vi "Process.vi"(8 "error in":errorcluster, 11 "StreamReader":refnum<class "StreamReader.lvclass">) -> (0 "error out":errorcluster, 3 "StreamReader out":refnum<class "StreamReader.lvclass">)   [LabVIEW 2016, in "StreamReader.lvclass"]
doc: "---------------------------------------------------------------\nJKI State Machine Objects™\nhttp://jki.net/state-machine-objects/\nCopyright (C) 2005-2015, JKI <info@jki.net>\nALL RIGHTS RESERVED"
uses:
  StreamReader.lvclass
  C:/Program Files/National Instruments/LabVIEW 2016/vi.lib/JKI/JKI SMO/SMO/SMO.lvclass
  <vilib>/JKI/JKI SMO/SMO/Typedefs/Parent Call--Enum.ctl
  <vilib>/JKI/JKI SMO/SMO/SMO.lvclass
  <resource>/objmgr/ni.dex.rc
panel:
  in  "start":bool
  in  "stop":bool
  out "full URL":string
  in  "Target IP Address":string="localhost"
  out "Signals Graph":waveform(dbl)[](graph)=[{"t0"=timestamp(3565974471.4961195 s since 1904-01-01), "dt"=1.0, "Y"=array[6023 elements], "attributes"=variant("NI_ChannelName"=variant(string "Dev2/ai0"), "NI_UnitDescription"=variant(string "Volts"))}, {"t0"=timestamp(3565974471.4961195 s since 1904-01-01), "dt"=1.0, "Y"=array[6023 elements], "attributes"=variant("NI_ChannelName"=variant(string "Dev2/ai1"), "NI_UnitDescription"=variant(string "Volts"))}, {"t0"=timestamp(3565974471.4961195 s since 1904-01-01), "dt"=1.0, "Y"=array[6023 elements], "attributes"=variant("NI_ChannelName"=variant(string "Dev2/ai2"), "NI_UnitDescription"=variant(string "Volts"))}, {"t0"=timestamp(3565974471.4961195 s since 1904-01-01), "dt"=1.0, "Y"=array[6023 elements], "attributes"=variant("NI_ChannelName"=variant(string "Dev2/ai3"), "NI_UnitDescription"=variant(string "Volts"))}, {"t0"=timestamp(3565974471.554943 s since 1904-01-01), "dt"=1.0, "Y"=array[6023 elements], "attributes"=variant("NI_ChannelName"=variant(string "Dev2/ai0"), "NI_UnitDescription"=variant(string "Volts"))}, {"t0"=timestamp(3565974471.554943 s since 1904-01-01), "dt"=1.0, "Y"=array[6023 elements], "attributes"=variant("NI_ChannelName"=variant(string "Dev2/ai1"), "NI_UnitDescription"=variant(string "Volts"))}]
  out "Available Elements to Read":i32
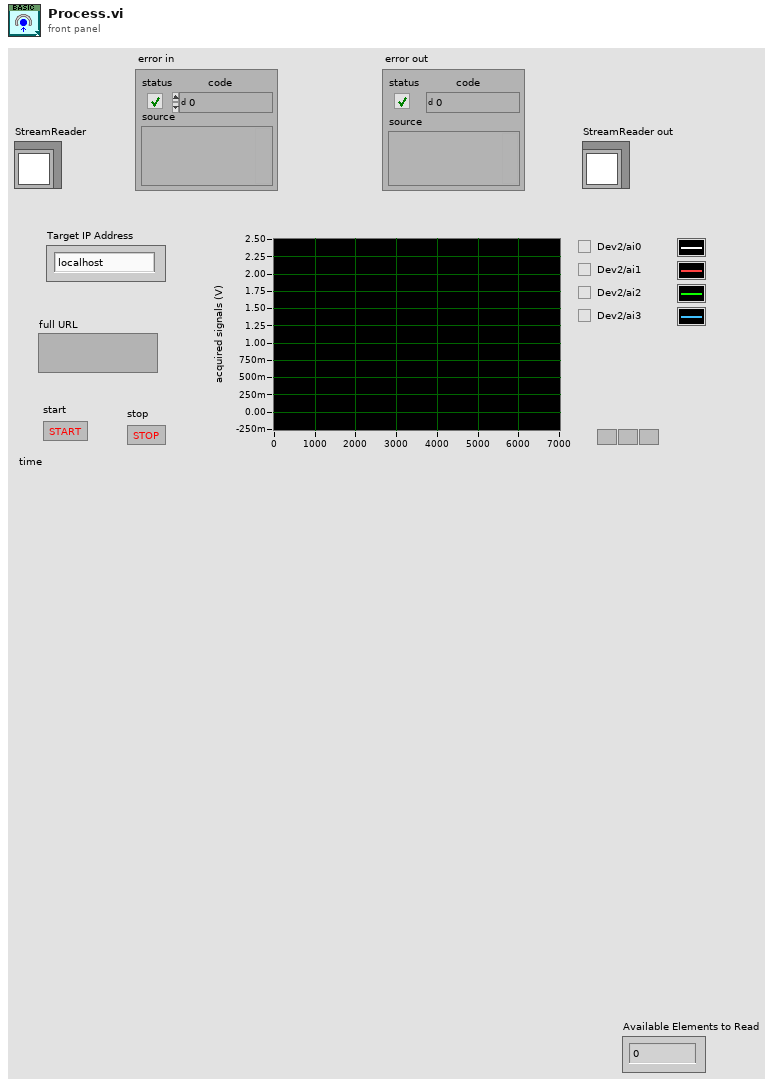
[diagram p1: front panel]
types:
  T1 = typedef "SMO.lvclass/Parent Call--Enum.ctl" = enum16{"Allows parent to run", "Does not request parent to run"}
  T2 = enum32{"invalid app kind", "Development System", "Run Time System", "Student Edition", "Embedded LabVIEW", "Evaluation", "Custom"}
  T3 = enum32{"Invalid", "Standard", "Closed", "Hidden", "Minimized", "Maximized"}
  T4 = enum32{"Bad", "Idle", "Run top level", "Running"}
  T5 = cluster{"Core":cluster{"Current VI Reference":refnum<vi>, "Close Panel on Exit?":bool, "error":errorcluster}, "Self Reference":refnum<class "StreamReader.lvclass">, "Your string data":string, "reader endpoint":refnum<k21>}
  T6 = cluster{"Current VI Reference":refnum<vi>, "Close Panel on Exit?":bool, "error":errorcluster}
  T7 = typedef "SMO.lvclass/Protected Events.ctl" = cluster{"StopProcesses":refnum<user-event>, "AbortProcesses":refnum<user-event>, "Config Changed":refnum<user-event>, "Dependency":refnum<user-event>}
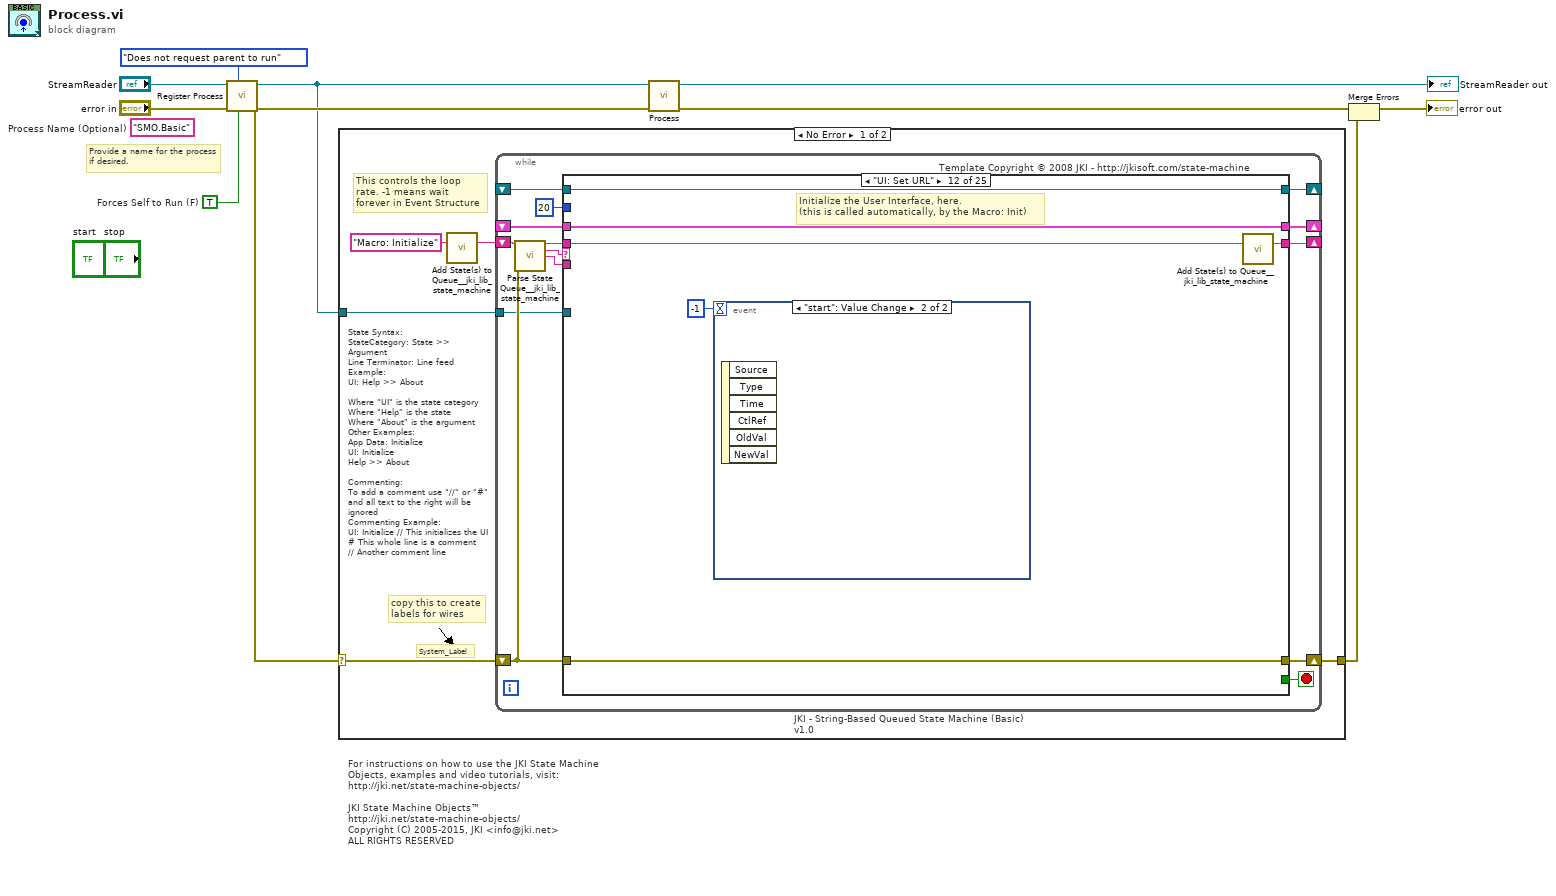
[diagram p0: block diagram]
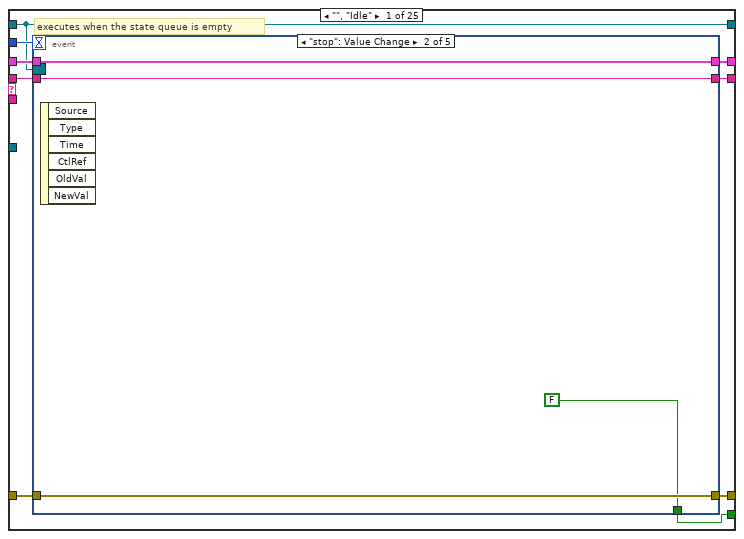
[diagram p2: hidden frame]
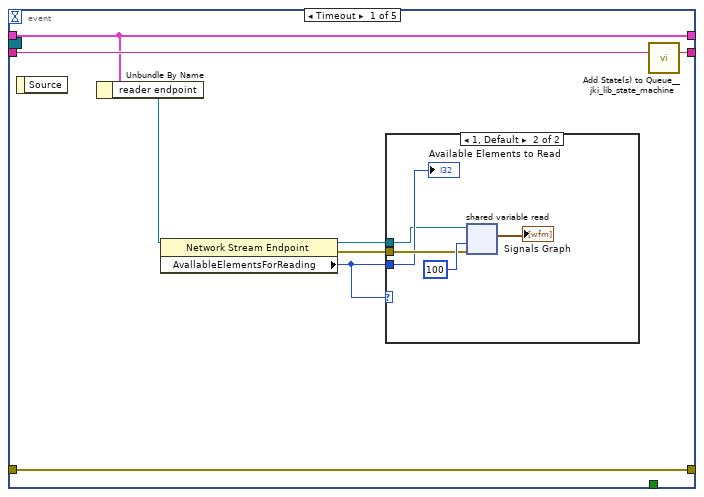
[diagram p3: hidden frame]
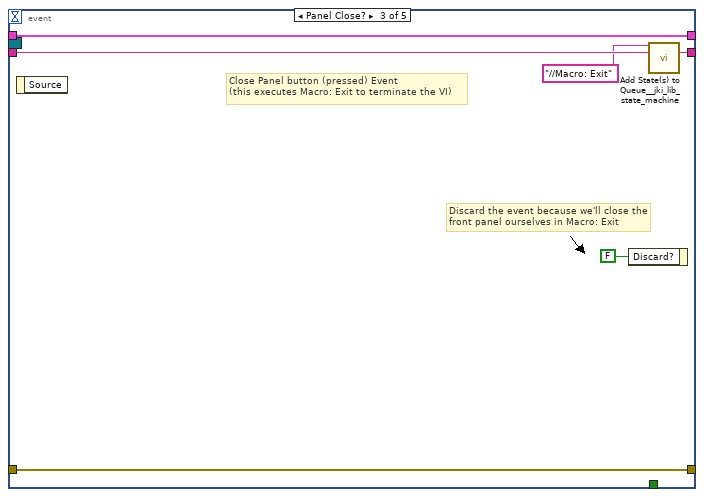
[diagram p5: hidden frame]
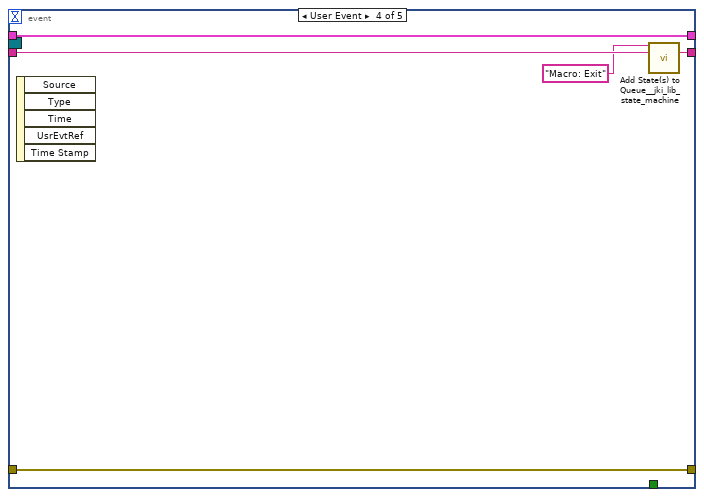
[diagram p6: hidden frame]
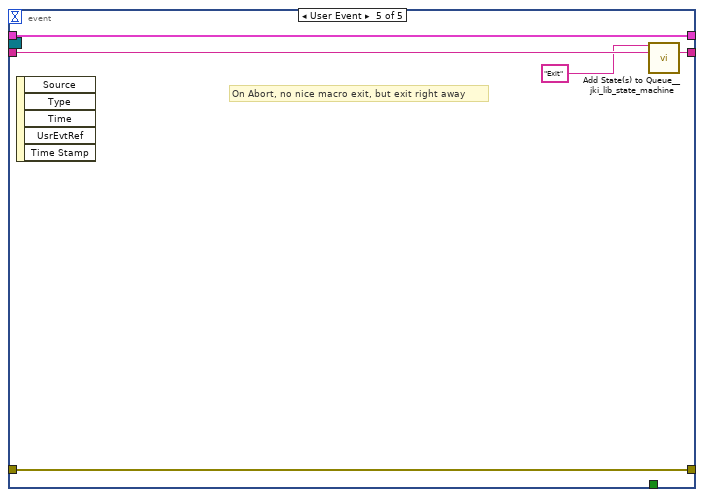
[diagram p7: hidden frame]
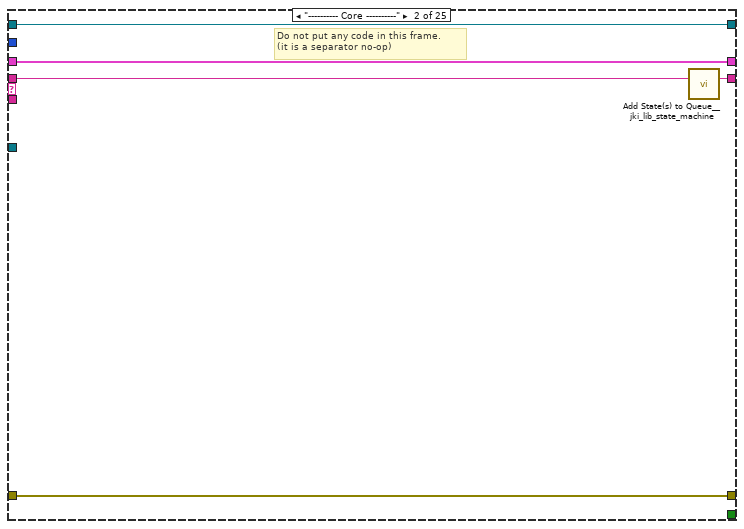
[diagram p8: hidden frame]
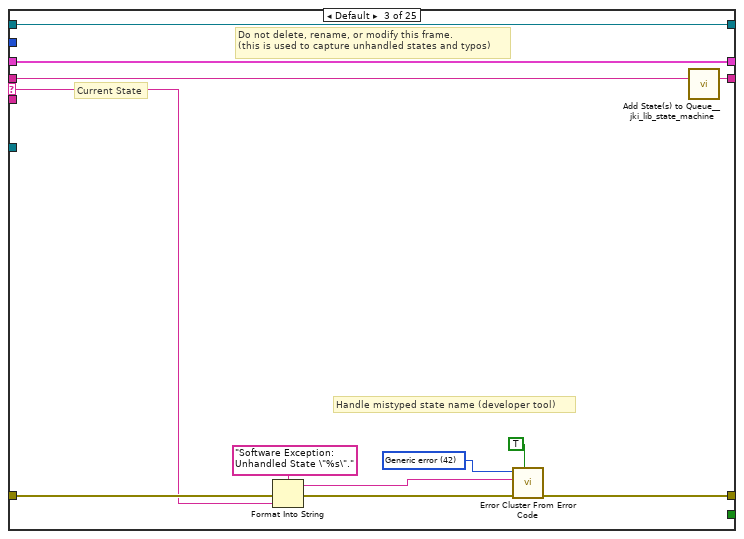
[diagram p9: hidden frame]
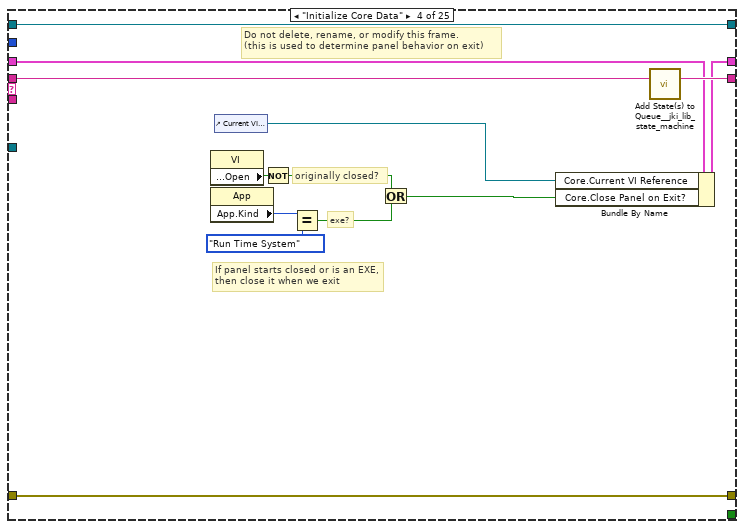
[diagram p10: hidden frame]
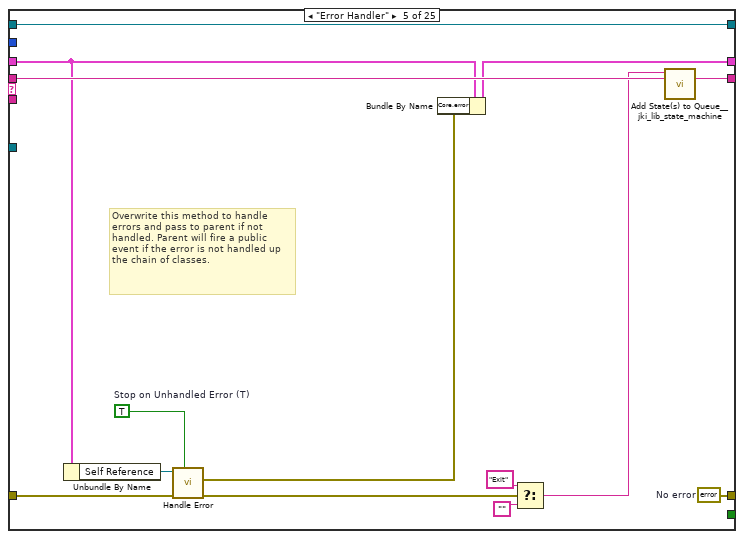
[diagram p11: hidden frame]
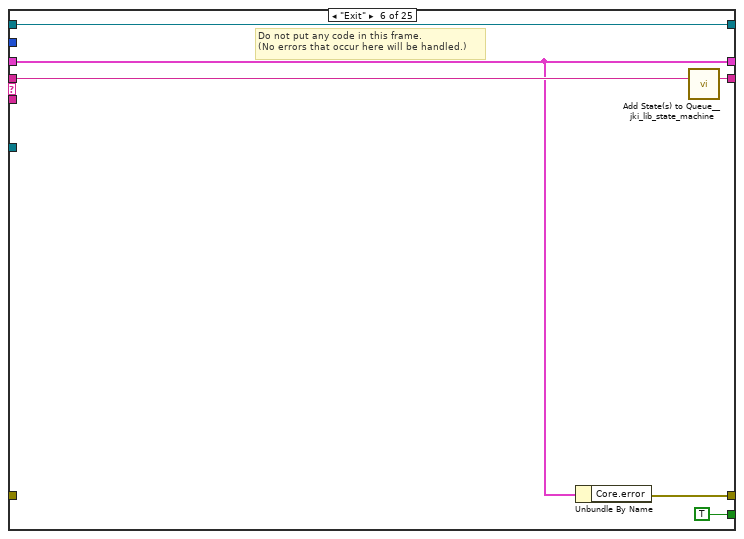
[diagram p12: hidden frame]
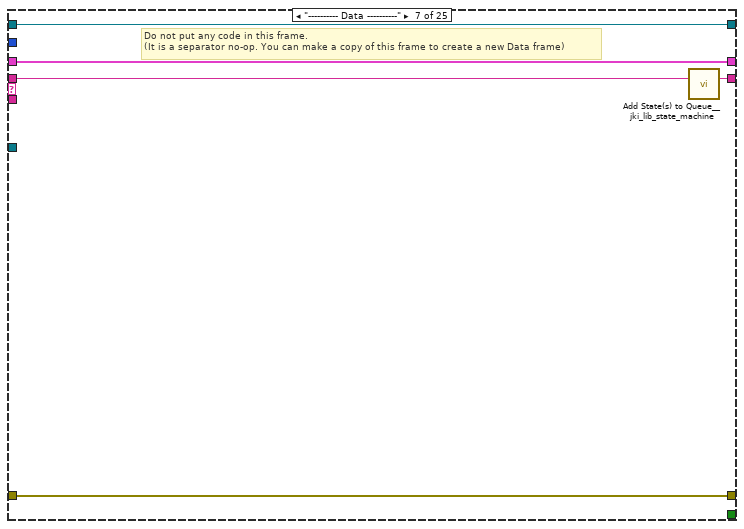
[diagram p13: hidden frame]
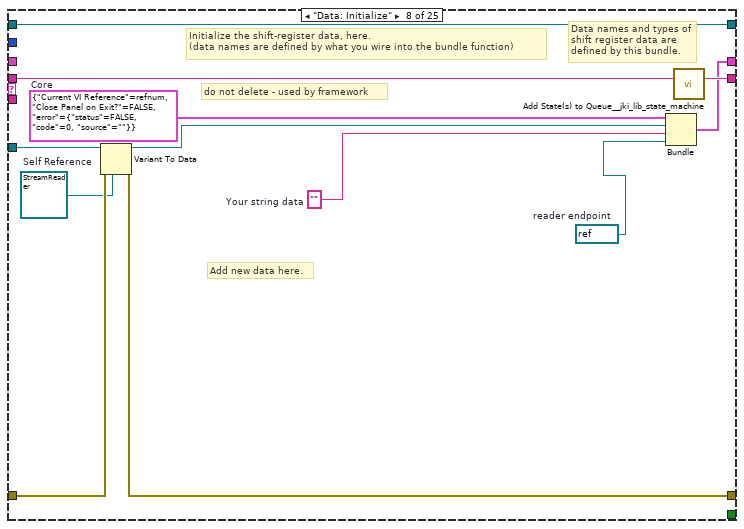
[diagram p14: hidden frame]
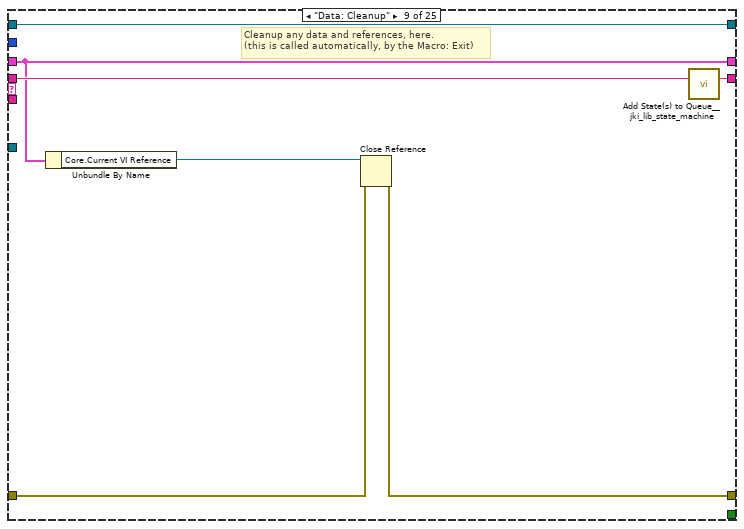
[diagram p15: hidden frame]
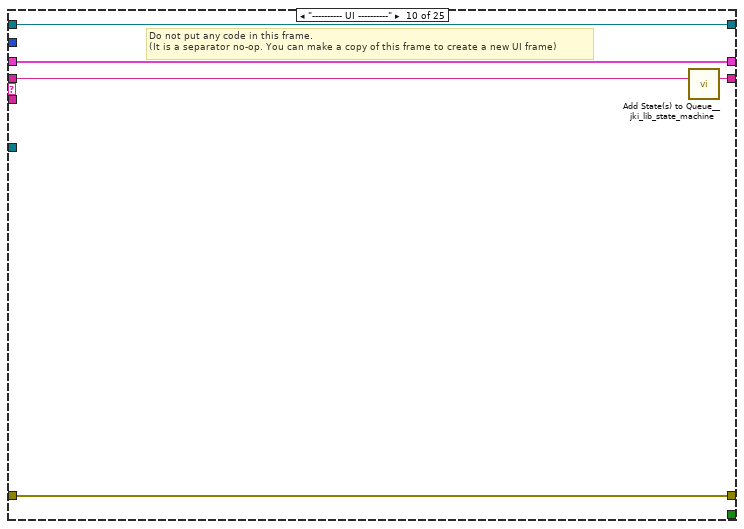
[diagram p16: hidden frame]
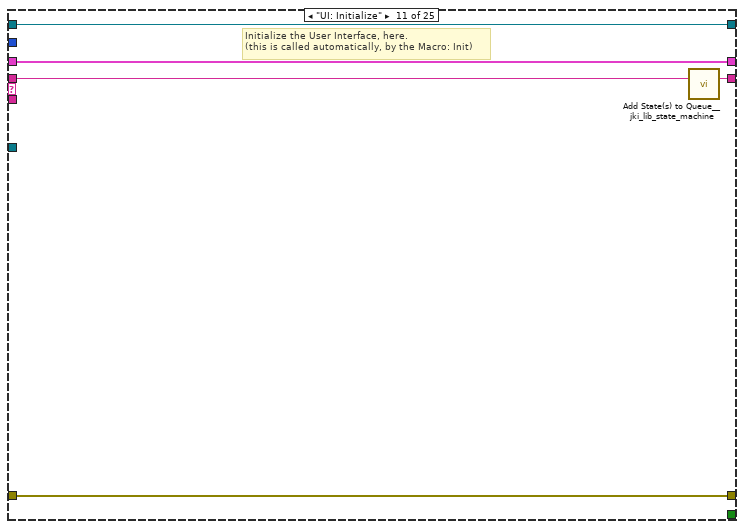
[diagram p17: hidden frame]
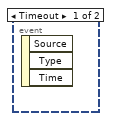
[diagram p18: hidden frame]
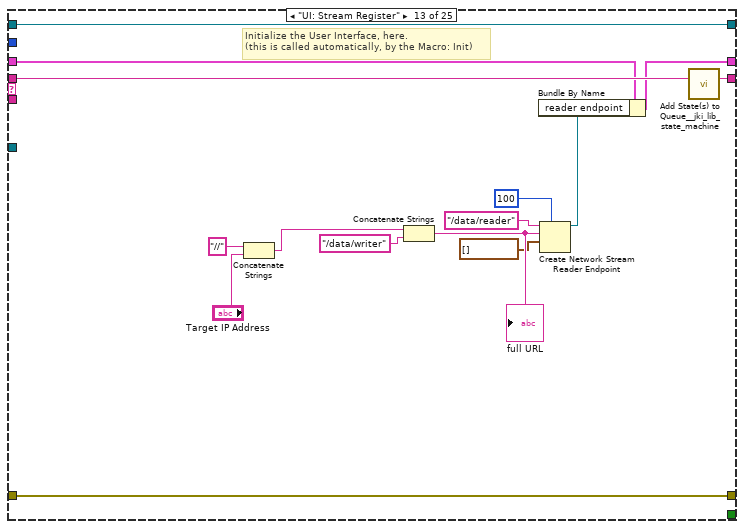
[diagram p19: hidden frame]
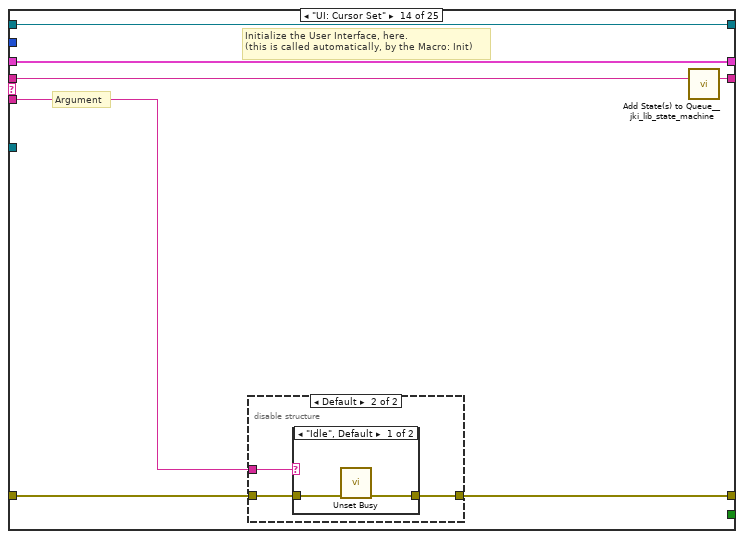
[diagram p20: hidden frame]
diagram:
  w1 = TRUE  # Forces Self to Run (F)
  (unwired) "SMO.Basic"  # Process Name (Optional)
  # "Provide a name for the process\nif desired."
  # "For instructions on how to use the JKI State Machine Objects, examples and video tutorials, visit:\nhttp://jki.net/state-machine-objects/\n\nJKI State Machine Objects™\nhttp://jki.net/state-machine-objects/\nCopyright (C) 2005-2015, JKI <info@jki.net>\nALL RIGHTS RESERVED"
  n1 = call <vilib>:"Register Process.vi"("Forces Self to Run (F)"=w1, "Parent Call"=Parent_Call--Enum."Does not request parent to run", "error in (no error)"="error in", "SMO"="StreamReader") -> ("error out"=w7:errorcluster, "SMO out"=w6:refnum<class "StreamReader.lvclass">)  [unwired: 6 in]
  n2 = case shown="No Error" w7 {
    selector: w7 -> [w12 w310]
    tunnel: w6 -> [w13 _]
    tunnel: [w11 w310] -> w3
    frame No Error {
      # "State Syntax:\nStateCategory: State >> Argument\nLine Terminator: Line feed\nExample:\nUI: Help >> About\n\nWhere \"UI\" is the state category\nWhere \"Help\" is the state\nWhere \"About\" is the argument\nOther Examples:\nApp Data: Initialize\nUI: Initialize\nHelp >> About\n\nCommenting:\nTo add a comment use \"//\" or \"#\" and all text to the right will be ignored\nCommenting Example:\nUI: Initialize // This initializes the UI\n# This whole line is a comment\n// Another comment line"
      # "copy this to create labels for wires"
      # "This controls the loop rate. -1 means wait forever in Event Structure"
      # "System_Label"
      n3 = call <vilib>:"Add State(s) to Queue__jki_lib_state_machine.vi"("State(s) in (\"\")"="Macro: Initialize") -> ("States Out"=w15:string)  [unwired: 14 in]
      n4 = while "JKI - String-Based Queued State Machine (Basic) v1.0" {
        shift-right: [w22] -> _
        shift-left: _ -> [w21]
        shift-right: [w25] -> w11
        shift-left: w12 -> [w19]
        shift-right: [w24] -> _
        shift-left: w15 -> [w26]
        tunnel: w13 -> [w18]
        shift-right: [w17] -> _
        shift-left: _ -> [w16]
        stop <- w23 stop-if-true
        # "Template Copyright © 2008 JKI - http://jkisoft.com/state-machine"
        n5 = call <vilib>:"Parse State Queue__jki_lib_state_machine.vi"("State Queue"=w26, "Error In (no error)"=w19) -> ("Remaining States"=w28:string, "Current State"=w29:string, "Arguments"=w27:string)  [unwired: 11 in]
        n6 = case shown="\"UI: Set URL\"" w29 {
          selector: w29 -> [_ _ w78 _ _ _ _ _ _ _ _ _ _ _ _ _ _ _ _ _ _ _ _ _ _]
          tunnel: w28 -> [w38 w76 w82 w101 w115 w121 w126 w138 w145 w150 w155 w161 w176 w183 w199 w231 w245 w260 w265 w276 w281 w291 w297 w302 w309]
          tunnel: w27 -> [_ _ _ _ _ _ _ _ _ _ _ _ _ w177 w193 _ _ _ _ _ _ _ _ _ _]
          tunnel: w21 -> [w36 w73 w80 w92 w109 w117 w123 _ w140 w147 w151 w157 w166 w181 w195 w228 w241 w251 w262 w273 w278 w289 w295 w300 w305]
          tunnel: [w35 w74 w84 w98 w110 w116 w124 w133 w141 w148 w153 w159 w174 w178 w196 w229 w243 w258 w263 w267 w279 w284 w293 w298 w306] -> w25
          tunnel: w19 -> [w34 w74 w83 w98 w111 _ w124 w134 w142 w148 w153 w159 w174 w179 w197 w229 w243 w258 w263 w268 w279 w285 w293 w298 w306]
          tunnel: [w37 w75 w81 w100 w114 w120 w125 w137 w144 w149 w154 w160 w175 w182 w198 w230 w244 w259 w264 w275 w280 w290 w296 w301 w308] -> w24
          tunnel: [w30 _ _ _ _ TRUE _ _ _ _ _ _ _ _ _ _ _ _ _ _ _ _ _ _ _] -> w23
          tunnel: [w33 w73 w80 w99 w108 w117 w123 w136 w140 w147 w151 w157 w165 w181 w195 w228 w241 w251 w262 w273 w278 w289 w295 w300 w304] -> w22
          tunnel: 20 ("Timeout") -> [w32 _ _ _ _ _ _ _ _ _ _ _ _ _ _ _ _ _ _ _ _ _ _ _ _]
          tunnel: w18 -> [_ _ _ _ _ _ _ w131 _ _ _ _ _ _ _ _ _ _ _ _ _ _ _ _ _]
          tunnel: [w31 w72 w77 w89 w113 w118 w122 w129 w139 w146 w152 w158 w173 w180 w192 w227 w242 w252 w261 w274 w277 w288 w294 w299 w307] -> w17
          tunnel: w16 -> [w31 w72 w77 w89 w113 w118 w122 w129 w139 w146 w152 w158 w173 w180 w192 w227 w242 w252 w261 w274 w277 _ w294 w299 w307]
          frame "", "Idle" {
            # "executes when the state queue is empty"
            n7 = event shown="[1] \"stop\": Value Change" {
              selector: w31 -> [_ _ _ _ _]
              dyn-events: _ -> [_ _ _ _ _]
              timeout: w32 -> [_ _ _ _ _]
              tunnel: w38 -> [w46 w53 w61 w66 w71]
              tunnel: [w45 w53 w60 w65 w70] -> w37
              tunnel: w36 -> [w41 w54 w58 w63 w68]
              tunnel: [w44 w55 w59 w64 w69] -> w35
              tunnel: w34 -> [w44 w55 w59 w64 w69]
              tunnel: [w41 w54 w58 w63 w68] -> w33
              tunnel: [_ FALSE _ _ _] -> w30
              event Timeout {
                n8 = event-data() -> ()  [unwired: 1 in, 1 out]
                n9 = Unbundle By Name(w41) -> ("reader endpoint"=w40:refnum<k21>)
                n10 = property class="Network Stream Endpoint"(reference=w40) -> (reference out=w42:refnum<k21>, error out=w43:errorcluster, "AvallableElementsForReading"=w39:i32)  [unwired: 1 in]
                n11 = case shown="1, Default" w39 {
                  tunnel: w43 -> [_ w50]
                  tunnel: w39 -> [_ w49]
                  tunnel: w42 -> [_ w47]
                  frame 0 {
                  }
                  frame 1, Default {
                    n12 = shared-variable-read(w47, w50, 100 ("timeout ms")) -> (→"Signals Graph":waveform(dbl)[])  [unwired: 3 out]
                    "Available Elements to Read" <- w49
                  }
                }
                n13 = call <vilib>:"Add State(s) to Queue__jki_lib_state_machine.vi"("State(s) in (\"\")"=w46) -> ("States Out"=w45:string)  [unwired: 14 in]
              }
              event "stop": Value Change {
                n14 = event-data() -> ()  [unwired: 1 in, 6 out]
              }
              event Panel Close? {
                # "Discard the event because we'll close the front panel ourselves in Macro: Exit"
                # "Close Panel button (pressed) Event\n(this executes Macro: Exit to terminate the VI)"
                n15 = event-data() -> ()  [unwired: 1 in, 1 out]
                n16 = event-data("Discard?"=FALSE) -> ()  [unwired: 1 in, 1 out]
                n17 = call <vilib>:"Add State(s) to Queue__jki_lib_state_machine.vi"("State(s) in Front (\"\")"="//Macro: Exit", "State(s) in (\"\")"=w61) -> ("States Out"=w60:string)  [unwired: 13 in]
              }
              event User Event {
                n18 = event-data() -> ()  [unwired: 1 in, 5 out]
                n19 = call <vilib>:"Add State(s) to Queue__jki_lib_state_machine.vi"("State(s) in Front (\"\")"="Macro: Exit", "State(s) in (\"\")"=w66) -> ("States Out"=w65:string)  [unwired: 13 in]
              }
              event User Event {
                # "On Abort, no nice macro exit, but exit right away"
                n20 = event-data() -> ()  [unwired: 1 in, 5 out]
                n21 = call <vilib>:"Add State(s) to Queue__jki_lib_state_machine.vi"("State(s) in Front (\"\")"="Exit", "State(s) in (\"\")"=w71) -> ("States Out"=w70:string)  [unwired: 13 in]
              }
            }
          }
          frame "---------- Core ----------" {
            # "Do not put any code in this frame.\n(it is a separator no-op)"
            n22 = call <vilib>:"Add State(s) to Queue__jki_lib_state_machine.vi"("State(s) in (\"\")"=w76) -> ("States Out"=w75:string)  [unwired: 14 in]
          }
          frame Default {
            w87 = 42 items=["No error", "Argument error", "Memory is full", "Out of zone", "End of file", "File already open", "Generic file I/O error", "File not found", "File permission error", "Disk is full", "Duplicate path", "Too many files open", "System feature not enabled", "Resource file not found", "Cannot add resource", "Resource not found", "Image not found", "Image memory error", "Pen does not exist", "Config type invalid", "Config token not found", "Config parse error", "Config memory error", "Bad external code format", "Bad external code offset", "External code not present", "Null window", "Destroy window error", "Null menu", "Print aborted", "Bad print record", "Print driver error", "Windows error during printing", "Memory error during printing", "Print dialog error", "Generic print error", "Invalid device refnum", "Device not found", "Device parameter error", "Device unit error", "Cannot open device", "Device call aborted", "Generic error", "Cancelled by user", "Object ID too low", "Object ID too high", "Object not in heap", "Unknown heap", "Unknown object (invalid DefProc)", "Unknown object (DefProc not in table)", "Message out of range", "Invalid (null) method", "Unknown message", "Manager call not supported", "Bad address", "Network operation in progress", "Network operation timed out", "Connection is busy", "Network attribute not supported", "Network error", "Address in use", "System out of memory", "Connection aborted", "Connection refused", "Not connected", "Already connected", "Connection closed", "Initialization error (interapplication manager)", "Bad occurrence", "Wait on unbound occurrence handler", "Occurrence queue overflow", "Datalog type conflict", "Unused", "Unrecognized type (interapplication manager)", "Memory corrupt", "Failed to make temporary DLL", "Old CIN version", "Drag socket not found", "Failed to load drop-object", "Failed to register OLE object", "Failed to release OLE object", "Format specifier type mismatch", "Unknown format specifier", "Too few format specifiers", "Too many format specifiers", "Scan failed", "Newer CIN version", "Error converting to variant", "Runtime menu error", "Password tampered", "Variant attribute not found", "Incompatible variant data type", "Event data is not available", "Event Store is not present", "Occurrence is not found", "Event Queue is not created", "Event info is not available", "Refnum passed is NULL", "Error retrieving Class GUID", "Error retrieving CoClass GUID", "Error retrieving TypeLib GUID.", "Bad built application magic bytes.", "Specific driver is different from the specific driver associated with the Logical Name.", "There is no session opened to the class driver.", "Max Error", "MAX - Error with config objects", "MAX - Error loading configuration", "MAX - Group not supported"]
            # "Current State"
            # "Do not delete, rename, or modify this frame.\n(this is used to capture unhandled states and typos)"
            # "Handle mistyped state name (developer tool)"
            n23 = Format Into String(format string="Software Exception: Unhandled State \"%s\"." ("message"), error in=w83, w78) -> (resulting string=w86:string, error out=w85:errorcluster)  [unwired: 1 in]
            n24 = call <vilib>:"Error Cluster From Error Code.vi"("show call chain? (False)"=TRUE, "error in (no error)"=w85, "error message (\"\")"=w86, "error code (0)"=w87) -> ("error out"=w84:errorcluster)  [unwired: 5 in]
            n25 = call <vilib>:"Add State(s) to Queue__jki_lib_state_machine.vi"("State(s) in (\"\")"=w82) -> ("States Out"=w81:string)  [unwired: 14 in]
          }
          frame "Initialize Core Data" {
            # "Do not delete, rename, or modify this frame.\n(this is used to determine panel behavior on exit)"
            # "originally closed?"
            # "exe?"
            # "If panel starts closed or is an EXE, then close it when we exit"
            n26 = property class="VI"() -> ("Front Panel.Open"=w97:bool)  [unwired: 2 in, 2 out]
            n27 = property class="App"() -> ("App.Kind"=w96:T2)  [unwired: 2 in, 2 out]
            n28 = control-ref of="Current VI Reference"() -> (w90:refnum<vi>)
            n29 = Not(x=w97) -> (.not. x?=w94:bool)
            n30 = Equal?(x=w96, y=T2."Run Time System" ("Application:Kind")) -> (x = y?=w93:bool)
            n31 = Or(x=w94, y=w93) -> (x .or. y?=w91:bool)
            n32 = Bundle By Name(cluster=w92, "Core.Current VI Reference"=w90, "Core.Close Panel on Exit?"=w91) -> (w99:T5)
            n33 = call <vilib>:"Add State(s) to Queue__jki_lib_state_machine.vi"("State(s) in (\"\")"=w101) -> ("States Out"=w100:string)  [unwired: 14 in]
          }
          frame "Error Handler" {
            w102 = TRUE  # Stop on Unhandled Error (T)
            w110 = errorcluster {"status"=FALSE, "code"=0, "source"=""}  # No error
            # "Overwrite this method to handle errors and pass to parent if not handled. Parent will fire a public event if the error is not handled up the chain of classes."
            n34 = Unbundle By Name(w109) -> ("Self Reference"=w112:refnum<class "StreamReader.lvclass">)
            n35 = call-dynamic "Handle Error.vi"("Stop on Unhandled Error (T)"=w102, "error in"=w111, "SMO"=w112) -> ("handling error"=w103:errorcluster, "Unhandled error"=w106:errorcluster)  [unwired: 6 in, 1 out]
            n36 = Bundle By Name(cluster=w109, "Core.error"=w106) -> (w108:T5)
            n37 = Select(t="Exit", s=w103, f="") -> (s? t:f=w107:string)
            n38 = call <vilib>:"Add State(s) to Queue__jki_lib_state_machine.vi"("State(s) in Front (\"\")"=w107, "State(s) in (\"\")"=w115) -> ("States Out"=w114:string)  [unwired: 13 in]
          }
          frame "Exit" {
            # "Do not put any code in this frame.\n(No errors that occur here will be handled.)"
            n39 = Unbundle By Name(w117) -> ("Core.error"=w116:errorcluster)
            n40 = call <vilib>:"Add State(s) to Queue__jki_lib_state_machine.vi"("State(s) in (\"\")"=w121) -> ("States Out"=w120:string)  [unwired: 14 in]
          }
          frame "---------- Data ----------" {
            # "Do not put any code in this frame.\n(It is a separator no-op. You can make a copy of this frame to create a new Data frame)"
            n41 = call <vilib>:"Add State(s) to Queue__jki_lib_state_machine.vi"("State(s) in (\"\")"=w126) -> ("States Out"=w125:string)  [unwired: 14 in]
          }
          frame "Data: Initialize" {
            w127 = refnum<k21> refnum  # reader endpoint
            w128 = T6 {"Current VI Reference"=refnum, "Close Panel on Exit?"=FALSE, "error"={"status"=FALSE, "code"=0, "source"=""}}  # Core
            w132 = refnum<class "StreamReader.lvclass"> refnum  # Self Reference
            w135 = ""  # Your string data
            # "do not delete - used by framework"
            # "Add new data here."
            # "Data names and types of shift register data are defined by this bundle."
            # "Initialize the shift-register data, here.\n(data names are defined by what you wire into the bundle function)"
            n42 = Variant To Data(error in=w134, type=w132, Variant=w131) -> (data=w130:refnum<class "StreamReader.lvclass">, error out=w133:errorcluster)
            n43 = Bundle("Core"=w128, "Self Reference"=w130, "Your string data"=w135, "reader endpoint"=w127) -> (w136:T5)  [unwired: 1 in]
            n44 = call <vilib>:"Add State(s) to Queue__jki_lib_state_machine.vi"("State(s) in (\"\")"=w138) -> ("States Out"=w137:string)  [unwired: 14 in]
          }
          frame "Data: Cleanup" {
            # "Cleanup any data and references, here.\n(this is called automatically, by the Macro: Exit)"
            n45 = Unbundle By Name(w140) -> ("Core.Current VI Reference"=w143:refnum<vi>)
            n46 = Close Reference(reference=w143, error in (no error)=w142) -> (error out=w141:errorcluster)
            n47 = call <vilib>:"Add State(s) to Queue__jki_lib_state_machine.vi"("State(s) in (\"\")"=w145) -> ("States Out"=w144:string)  [unwired: 14 in]
          }
          frame "---------- UI ----------" {
            # "Do not put any code in this frame.\n(It is a separator no-op. You can make a copy of this frame to create a new UI frame)"
            n48 = call <vilib>:"Add State(s) to Queue__jki_lib_state_machine.vi"("State(s) in (\"\")"=w150) -> ("States Out"=w149:string)  [unwired: 14 in]
          }
          frame "UI: Initialize" {
            # "Initialize the User Interface, here.\n(this is called automatically, by the Macro: Init)"
            n49 = call <vilib>:"Add State(s) to Queue__jki_lib_state_machine.vi"("State(s) in (\"\")"=w155) -> ("States Out"=w154:string)  [unwired: 14 in]
          }
          frame "UI: Set URL" {
            # "Initialize the User Interface, here.\n(this is called automatically, by the Macro: Init)"
            n50 = event shown="[1] \"start\": Value Change" {
              selector: _ -> [_ _]
              dyn-events: _ -> [_ _]
              timeout: -1 -> [_ _]
              event Timeout {
                n51 = event-data() -> ()  [unwired: 1 in, 3 out]
              }
              event "start": Value Change {
                n52 = event-data() -> ()  [unwired: 1 in, 6 out]
              }
            }
            n53 = call <vilib>:"Add State(s) to Queue__jki_lib_state_machine.vi"("State(s) in (\"\")"=w161) -> ("States Out"=w160:string)  [unwired: 14 in]
          }
          frame "UI: Stream Register" {
            # "Initialize the User Interface, here.\n(this is called automatically, by the Macro: Init)"
            n54 = Concatenate Strings("//" ("reader url"), "Target IP Address") -> (w162:string)
            n55 = Concatenate Strings(w162, "/data/writer" ("reader url")) -> (w170:string)
            "full URL" <- w170
            n56 = Create Network Stream Reader Endpoint(7:100 ("reader buffer size"), 9:waveform(dbl)[] [], 10:w170, 11:"/data/reader" ("writer name")) -> (3:w167:refnum<k21>)  [unwired: 3 in, 1 out]
            n57 = Bundle By Name(cluster=w166, "reader endpoint"=w167) -> (w165:T5)
            n58 = call <vilib>:"Add State(s) to Queue__jki_lib_state_machine.vi"("State(s) in (\"\")"=w176) -> ("States Out"=w175:string)  [unwired: 14 in]
          }
          frame "UI: Cursor Set" {
            # "Argument"
            # "Initialize the User Interface, here.\n(this is called automatically, by the Macro: Init)"
            n59 = disable-structure shown="Default" {
              disable-tunnel: w179 -> [w184 w187]
              disable-tunnel: [w184 w186] -> w178
              disable-tunnel: w177 -> [_ w185]
              frame condition #0 {
              }
              frame condition #1 (active) {
                n60 = case shown="\"Idle\", Default" w185 {
                  tunnel: w187 -> [w189 w191]
                  tunnel: [w188 w190] -> w186
                  frame "Idle", Default {
                    n61 = call <vilib>:"Unset Busy.vi"("error in (no error)"=w189) -> ("error out"=w188:errorcluster)  [unwired: 10 in]
                  }
                  frame "Busy" {
                    n62 = call <vilib>:"Set Busy.vi"("error in (no error)"=w191) -> ("error out"=w190:errorcluster)  [unwired: 9 in, 1 out]
                  }
                }
              }
            }
            n63 = call <vilib>:"Add State(s) to Queue__jki_lib_state_machine.vi"("State(s) in (\"\")"=w183) -> ("States Out"=w182:string)  [unwired: 14 in]
          }
          frame "UI: Front Panel State" {
            # "Argument"
            # "Set Front Panel Open or Closed\n(Usage: \"UI: Front Panel State >> Open|Close\")"
            n64 = Unbundle By Name(w195) -> ("Core.Current VI Reference"=w194:refnum<vi>)
            n65 = disable-structure shown="Default" {
              disable-tunnel: w197 -> [w203 w226]
              disable-tunnel: [w202 w226] -> w196
              disable-tunnel: w194 -> [w201 _]
              disable-tunnel: w193 -> [w200 _]
              frame condition #0 (active) {
                n66 = case shown="\"Close\"" w200 {
                  tunnel: w203 -> [w207 w220]
                  tunnel: [w209 w221] -> w202
                  tunnel: w201 -> [w208 w218]
                  frame "Open", Default {
                    n67 = property class="VI"(reference=w208, error in=w207) -> (reference out=w205:refnum<vi>, error out=w206:errorcluster, "FP.State"=w204:T3)
                    n68 = case shown="\"Closed\"" w204 {
                      tunnel: [w212 w215] -> w209
                      tunnel: w206 -> [w211 w215]
                      tunnel: w205 -> [w210 _]
                      frame "Closed" {
                        n69 = invoke class="VI" method="FP.Open"(reference=w210, error in=w211, "Activate"=TRUE, "State"=T3."Standard") -> (error out=w212:errorcluster)  [unwired: 1 in, 4 out]
                      }
                      frame Default {
                      }
                    }
                  }
                  frame "Close" {
                    n70 = property class="VI"(reference=w218, error in=w220) -> (reference out=w217:refnum<vi>, error out=w219:errorcluster, "FP.State"=w216:T3)
                    n71 = case shown="Default" w216 {
                      tunnel: [w222 w225] -> w221
                      tunnel: w219 -> [w222 w224]
                      tunnel: w217 -> [_ w223]
                      frame "Invalid", "Closed" {
                      }
                      frame Default {
                        n72 = invoke class="VI" method="FP.Close"(reference=w223, error in=w224) -> (error out=w225:errorcluster)  [unwired: 1 in, 2 out]
                      }
                    }
                  }
                }
              }
              frame condition #1 {
              }
            }
            n73 = call <vilib>:"Add State(s) to Queue__jki_lib_state_machine.vi"("State(s) in (\"\")"=w199) -> ("States Out"=w198:string)  [unwired: 14 in]
          }
          frame "---------- Macro ----------" {
            # "Do not put any code in this frame.\n(It is a separator no-op. You can make a copy of this frame to create a new Macro frame)"
            n74 = call <vilib>:"Add State(s) to Queue__jki_lib_state_machine.vi"("State(s) in (\"\")"=w231) -> ("States Out"=w230:string)  [unwired: 14 in]
          }
          frame "Macro: Initialize" {
            w236 = "UI: Initialize\nUI: Front Panel State >> Open\nUI: Set URL\nUI: Stream Register"  # UI: Initialize UI: Front Panel State >> Open UI: Set URL UI: Stream Register
            w232 = "Process: Sync"
            # "Initialization Macro\n(This is called once, when the VI starts)"
            n75 = control-ref of="This VI"() -> (w234:refnum<vi>)
            n76 = property class="VI"(reference=w234) -> ("Exec.State"=w233:T4)  [unwired: 1 in, 2 out]
            n77 = Equal?(x=w233, y=T4."Run top level") -> (x = y?=w239:bool)
            n78 = Select(t=w232, s=w239, f="") -> ()  [unwired: 1 out]
            n79 = call <vilib>:"Add State(s) to Queue__jki_lib_state_machine.vi"("State(s) in Front (\"\")"="Data: Initialize\nInitialize Core Data\nEvents: Register", "State(s) in (\"\")"=w232, "State(s) at Back (\"\")"=w236) -> ("States Out"=w235:string)  [unwired: 12 in]
            n80 = call <vilib>:"Add State(s) to Queue__jki_lib_state_machine.vi"("State(s) in Front (\"\")"=w235, "State(s) in (\"\")"=w245) -> ("States Out"=w244:string)  [unwired: 13 in]
          }
          frame "Macro: Exit" {
            # "Exit Macro\n(This is called once, when the VI exits)"
            n81 = Unbundle By Name(w251) -> ("Core.Close Panel on Exit?"=w257:bool, "reader endpoint"=w246:refnum<k21>)
            n82 = Destroy Stream Endpoint(11:w246) -> ()  [unwired: 1 in, 1 out]
            n83 = Select(t="//UI: Front Panel State >> Close", s=w257, f="") -> (s? t:f=w254:string)
            n84 = call <vilib>:"Add State(s) to Queue__jki_lib_state_machine.vi"("State(s) in Front (\"\")"="Data: Cleanup\nEvents: Unregister", "State(s) in (\"\")"="Process: Sync", "State(s) at Back (\"\")"="Exit") -> ("States Out"=w248:string)  [unwired: 12 in]
            n85 = call <vilib>:"Add State(s) to Queue__jki_lib_state_machine.vi"("State(s) in (\"\")"=w254, "State(s) at Back (\"\")"=w248) -> ("States Out"=w253:string)  [unwired: 13 in]
            n86 = call <vilib>:"Add State(s) to Queue__jki_lib_state_machine.vi"("State(s) in Front (\"\")"=w253, "State(s) in (\"\")"=w260) -> ("States Out"=w259:string)  [unwired: 13 in]
          }
          frame "---------- Process ----------" {
            # "Template Separator\n(You can make a copy of, or modify, this frame)"
            n87 = call <vilib>:"Add State(s) to Queue__jki_lib_state_machine.vi"("State(s) in (\"\")"=w265) -> ("States Out"=w264:string)  [unwired: 14 in]
          }
          frame "Process: Sync" {
            n88 = Unbundle By Name(w273) -> ("Self Reference"=w269:refnum<class "StreamReader.lvclass">)
            n89 = call <vilib>:"WaitOnProcessSync.vi"("error in (no error)"=w268, "SMO"=w269) -> ("error out"=w267:errorcluster, "Don't run?"=w272:bool)  [unwired: 7 in, 1 out]
            n90 = Select(t="Data: Cleanup\nEvents: Unregister\nExit", s=w272, f="") -> (s? t:f=w266:string)
            n91 = call <vilib>:"Add State(s) to Queue__jki_lib_state_machine.vi"("State(s) in Front (\"\")"=w266, "State(s) in (\"\")"=w276) -> ("States Out"=w275:string)  [unwired: 13 in]
          }
          frame "---------- Events ----------" {
            # "Template Separator\n(You can make a copy of, or modify, this frame)"
            n92 = call <vilib>:"Add State(s) to Queue__jki_lib_state_machine.vi"("State(s) in (\"\")"=w281) -> ("States Out"=w280:string)  [unwired: 14 in]
          }
          frame "Events: Register" {
            # "Expand to add\nmore events"
            n93 = Unbundle By Name(w289) -> ("Self Reference"=w286:refnum<class "StreamReader.lvclass">)
            n94 = call <vilib>:"GetProtectedEvents.vi"("SMO"=w286) -> ("error out"=w282:errorcluster, "SMO Protected Events"=w287:T7)  [unwired: 8 in, 1 out]
            n95 = register-events(w287) -> (reference out=w288:refnum<event-registration>, error out=w283:errorcluster)  [unwired: 2 in]
            n96 = Merge Errors(w285, w283, w282) -> (w284:errorcluster)
            n97 = call <vilib>:"Add State(s) to Queue__jki_lib_state_machine.vi"("State(s) in (\"\")"=w291) -> ("States Out"=w290:string)  [unwired: 14 in]
          }
          frame "Events: Unregister" {
            n98 = Unregister For Events(event registration refnum=w294, error in=w293) -> (error out=w292:errorcluster)
            n99 = call <vilib>:"Clear Errors.vi"("error in (no error)"=w292) -> ()  [unwired: 5 in, 2 out]
            n100 = call <vilib>:"Add State(s) to Queue__jki_lib_state_machine.vi"("State(s) in (\"\")"=w297) -> ("States Out"=w296:string)  [unwired: 14 in]
          }
          frame "---------- Action ----------" {
            n101 = call <vilib>:"Add State(s) to Queue__jki_lib_state_machine.vi"("State(s) in (\"\")"=w302) -> ("States Out"=w301:string)  [unwired: 14 in]
          }
          frame "Action: Template" {
            n102 = Unbundle By Name(w305) -> ("Self Reference"=w303:refnum<class "StreamReader.lvclass">)
            n103 = Bundle By Name(cluster=w305, "Self Reference"=w303) -> (w304:T5)
            n104 = call <vilib>:"Add State(s) to Queue__jki_lib_state_machine.vi"("State(s) in (\"\")"=w309) -> ("States Out"=w308:string)  [unwired: 14 in]
          }
        }
      }
    }
    frame Error {
    }
  }
  n105 = call-parent "Process.vi"("error in"=w7, "SMO"=w6) -> ("error out"=w4:errorcluster, "SMO out"=→"StreamReader out":refnum<class "StreamReader.lvclass">)  [unwired: 8 in]
  n106 = Merge Errors(w4, w3) -> (→"error out":errorcluster)
